vi "PicoScope3000aExampleRapidBlockBulk.vi"() -> ()   [LabVIEW 2016]
uses:
  PicoScope3000aLib/PicoScope3000aAnalogChannelSettings.ctl
panel:
  in  "Trigger Settings":T1={"Trigger Enabled"=FALSE, "Trigger Source"=enum."Channel A", "Trigger Threshold (volts)"=0.0, "Trigger Direction"=2, "Trigger Delay (samples)"=0, "Auto Trigger Time (ms)"=1000} {"Trigger Direction" items=["Above", "Below", "Rising", "Falling", "Rising or Falling"]}
  out "USB 3.0 device on non-USB 3.0 Port":bool=TRUE
  out "USB Powered":bool=TRUE
  in  "Use Serial number":bool
  in  "Batch/Serial":string
  out "Channel A":T2(graph)
  out "Properties Panel":T3 {"Max Total Capture Time Available (sec)" format="%.3p"; "Sample Frequency" format="%.3p"; "Sample Rate" format="%.3p"; "Max Samples Available" format="%.3p"; "Total Capture Time (sec)" format="%.3p"}
  out "Device Info":T4
  in  "Number of Segments":u32=10
  in  "Channel A Settings":T5={"Enabled"=TRUE, "Coupling"=1, "Range"=6, "Analogue Offset"=0.0, "Bandwidth Limit"=0} {"Bandwidth Limit" items=["Full", "20MHz"]; "Range" items=["10 mV", "20 mV", "50 mV", "100 mV", "200 mV", "500 mV", "1 V", "2 V", "5 V", "10 V", "20 V", "50 V ", "100 V"]; "Coupling" items=["AC", "DC"]}
  in  "Rapid Block Bulk Acquisition Settings":T6={"preTriggerSamples"=0, "postTriggerSamples"=10000, "timebase"=2, "Down-Sample Mode"=0, "Down Sample Ratio"=1, "Four Channel Device"=FALSE} {"Down Sample Ratio" min=1 step=1; "Down-Sample Mode" items=["None"=0, "Aggregate"=1, "Decimate"=2, "Average"=4]}
  out "Capture Complete":bool
  in  "Run":bool
  in  "Capture Index":i16 min=0
  in  "stop":bool
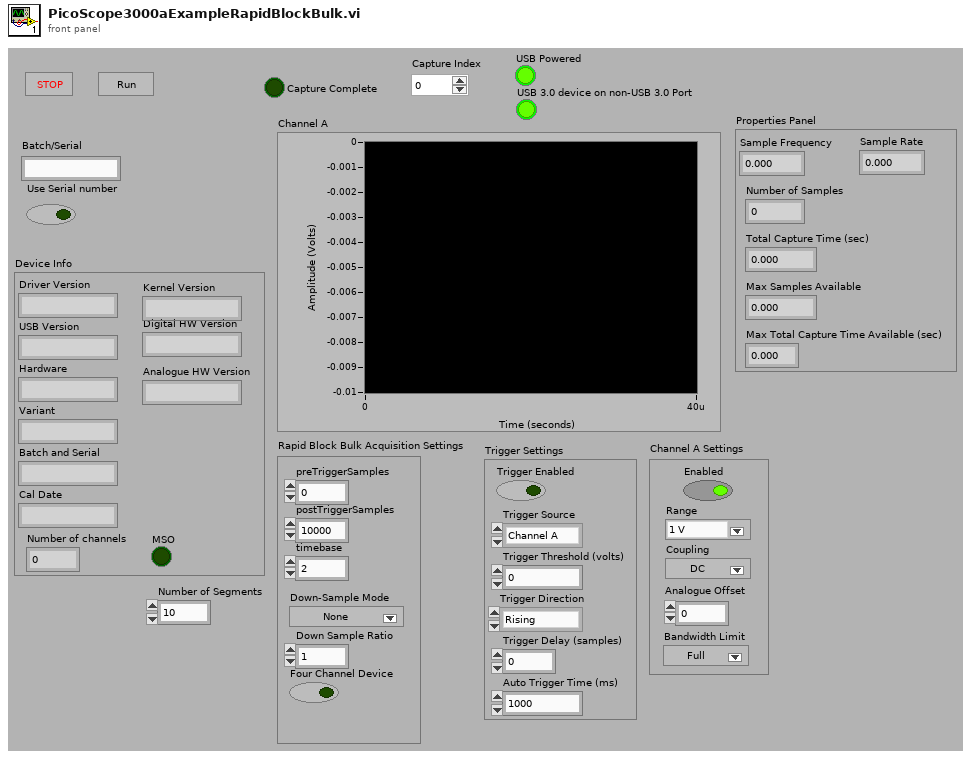
[diagram p1: front panel]
types:
  T1 = cluster{"Trigger Enabled":bool, "Trigger Source":enum32{"Channel A", "Channel B", "Channel C", "Channel D", "Ext."}, "Trigger Threshold (volts)":dbl, "Trigger Direction":u16, "Trigger Delay (samples)":u32, "Auto Trigger Time (ms)":i16}
  T2 = cluster{i32, "Sample Rate":sgl, "Data (Volts)":dbl[]}
  T3 = cluster{"Sample Frequency":sgl, "Sample Rate":sgl, "Max Samples Available":i32, "Number of Samples":u32, "Total Capture Time (sec) ":sgl, "Max Total Capture Time Available (sec)":sgl}
  T4 = cluster{"Driver Version":string, "USB Version":string, "Hardware":string, "Variant":string, "Batch and Serial":string, "Cal Date":string, "Kernel Version":string, "Digital HW Version":string, "Analogue HW Version":string, "MSO":bool, "Number of channels":i16}
  T5 = typedef "PicoScope3000aAnalogChannelSettings.ctl" = cluster{"Enabled":bool, "Coupling":u32, "Range":u32, "Analogue Offset":sgl, "Bandwidth Limit":u32}
  T6 = cluster{"preTriggerSamples":u32, "postTriggerSamples":u32, "timebase":u32, "Down-Sample Mode":i32, "Down Sample Ratio":u32, "Four Channel Device":bool}
  T7 = cluster{"preTriggerSamples":u32, "postTriggerSamples":u32, "timebase":u32, "Down-Sample Mode":i32, "Down Sample Ratio":u32}
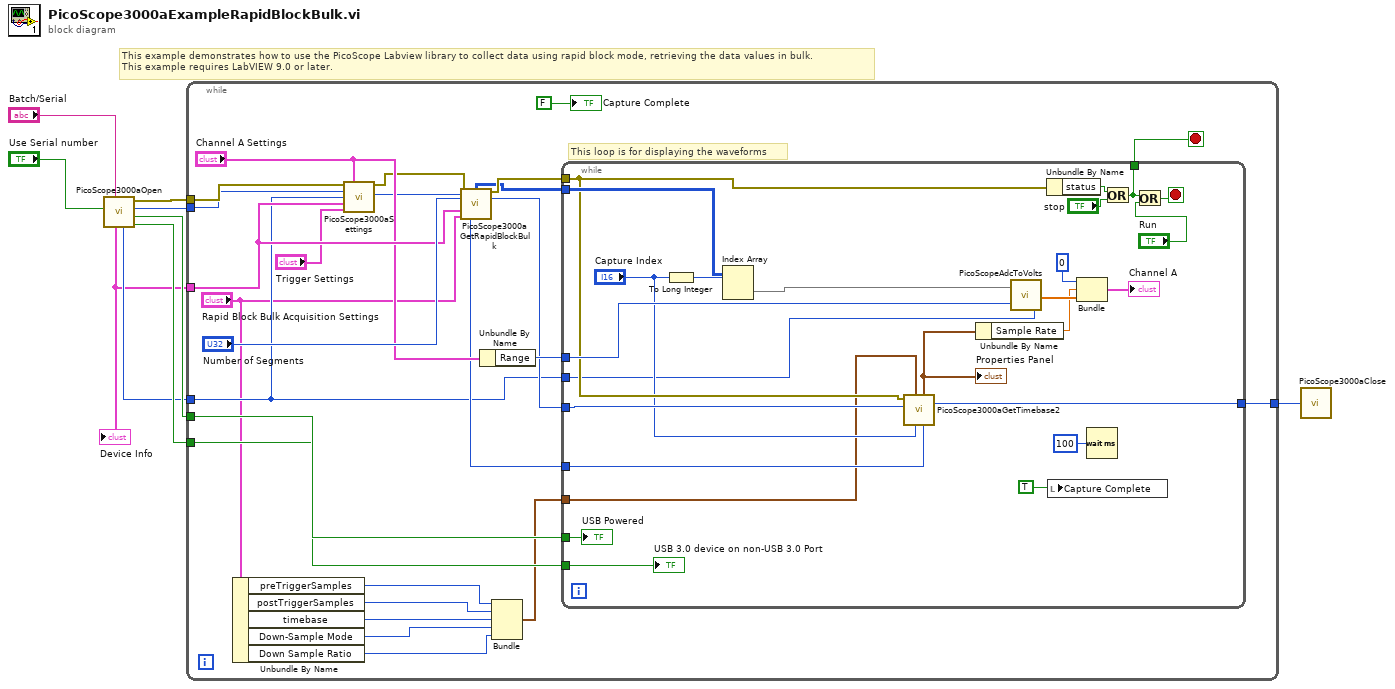
[diagram p0: block diagram]
diagram:
  # "This example demonstrates how to use the PicoScope Labview library to collect data using rapid block mode, retrieving the data values in bulk.\nThis example requires LabVIEW 9.0 or later."
  n1 = call "PicoScope3000aOpen.vi"("Batch/Serial"="Batch/Serial", "Use Serial number"="Use Serial number") -> ("USB 3.0 device on non-USB 3.0 Port"=w5:bool, "USB Powered"=w6:bool, "handle"=w7:i16, "error out"=w8:errorcluster, "Max ADC value"=w4:i16, "Device Info"=w3:T4)  [unwired: 4 in]
  "Device Info" <- w3
  n2 = while {
    tunnel: [w20] -> w9
    tunnel: w8 -> [w31]
    tunnel: w7 -> [w30]
    tunnel: w6 -> [w29]
    tunnel: w5 -> [w28]
    tunnel: w4 -> [w17]
    tunnel: w3 -> [w26]
    stop <- w35 stop-if-true
    # "This loop is for displaying the waveforms"
    n3 = Unbundle By Name("Rapid Block Bulk Acquisition Settings") -> ("preTriggerSamples"=w23:u32, "postTriggerSamples"=w22:u32, "timebase"=w21:u32, "Down-Sample Mode"=w14:i32, "Down Sample Ratio"=w13:u32)
    n4 = call "PicoScope3000aSettings.vi"("error in"=w31, "Channel A Settings"="Channel A Settings", "handle in"=w30, "Max_adc"=w17, "Device Info"=w26, "Trigger Settings"="Trigger Settings") -> ("error out"=w12:errorcluster, "handle out"=w11:i16)  [unwired: 7 in, 1 out]
    n5 = call "PicoScope3000aGetRapidBlockBulk.vi"("error in"=w12, "Number of Segments"="Number of Segments", "handle in"=w11, "Device Info"=w26, "Rapid Block Bulk Acquisition Settings"="Rapid Block Bulk Acquisition Settings") -> ("Channel A Buffer"=w32:i16[][], "error out"=w33:errorcluster, "handle out"=w19:i16, "Num samples"=w18:u32)  [unwired: 2 in, 5 out]
    n6 = Unbundle By Name("Channel A Settings") -> ("Range"=w24:u32)
    n7 = Bundle("preTriggerSamples"=w23, "postTriggerSamples"=w22, "timebase"=w21, "Down-Sample Mode"=w14, "Down Sample Ratio"=w13) -> (w16:T7)  [unwired: 1 in]
    n8 = while {
      tunnel: [w59] -> w35
      tunnel: w32 -> [w54]
      tunnel: w33 -> [w45]
      tunnel: w29 -> [w37]
      tunnel: w28 -> [w36]
      tunnel: w24 -> [w49]
      tunnel: [w46] -> w20
      tunnel: w19 -> [w44]
      tunnel: w18 -> [w41]
      tunnel: w17 -> [w40]
      tunnel: w16 -> [w39]
      stop <- w58 stop-if-true
      n9 = To Long Integer(number="Capture Index") -> (32bit integer=w43:i32)
      n10 = Index Array(array=w54, index (row)=w43) -> (element=w48:i16[])  [unwired: 1 in]
      n11 = call "PicoScope3000aGetTimebase2.vi"("Number of Samples"=w41, "Memory Segment"="Capture Index", "Acquisition Settings"=w39, "handle in"=w44, "error in (no error)"=w45) -> ("handle out"=w46:i16, "Properties Panel"=w47:T3)  [unwired: 4 in, 1 out]
      "Properties Panel" <- w47
      n12 = Unbundle By Name(w47) -> ("Sample Rate"=w50:sgl)
      n13 = call "PicoScopeAdcToVolts.vi"("Max_adc"=w40, "Range Index"=w49, "Data"=w48) -> ("Data"=w51:dbl[])
      n14 = Unbundle By Name(w45) -> ("status"=w55:bool)
      n15 = local write "Capture Complete"(TRUE ("Capture Complete")) -> ()
      n16 = Bundle(0, "Sample Rate"=w50, "Data"=w51) -> (→"Channel A":cluster{i32, "Sample Rate":sgl, "Data":dbl[]})  [unwired: 1 in]
      n17 = Wait (ms)(milliseconds to wait=u32 100) -> ()  [unwired: 1 out]
      n18 = Or(x=w55, y="stop") -> (x .or. y?=w59:bool)
      n19 = Or(x=w59, y="Run") -> (x .or. y?=w58:bool)
      "USB Powered" <- w37
      "USB 3.0 device on non-USB 3.0 Port" <- w36
    }
    "Capture Complete" <- FALSE ("Capture Complete")
  }
  n20 = call "PicoScope3000aClose.vi"("handle"=w9) -> ()
